vi "End Print.vi"(8 "error in (no error)":errorcluster, 11 "Stage Actor.lvlib:Stage.lvclass":refnum<class "Stage.lvclass">) -> (0 "error out":errorcluster, 3 "Actor out":refnum<class "Actor.lvclass">)   [LabVIEW 2018, in "Stage Actor.lvlib" / "Stage.lvclass"]
uses:
  Stage.lvclass
  <vilib>/ActorFramework/Actor/Actor.lvclass
  C:/Program Files/National Instruments/LabVIEW 2018/vi.lib/ActorFramework/Actor/Actor.lvclass
  Stage.lvclass/Stage.ctl
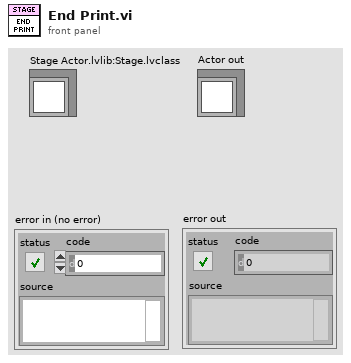
[diagram p1: front panel]
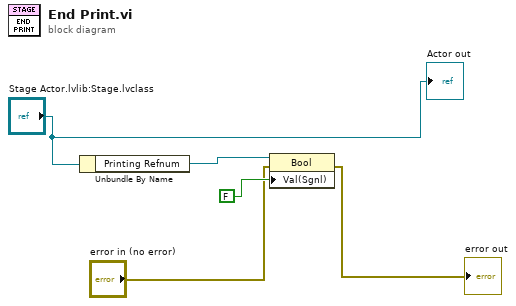
[diagram p0: block diagram]
diagram:
  n1 = Unbundle By Name("Stage Actor.lvlib:Stage.lvclass") -> ("Printing Refnum"=w5:refnum<vi>)
  n2 = property class="Bool"(reference=w5, error in="error in (no error)", "Val(Sgnl)"=FALSE) -> (error out=→"error out":errorcluster)  [unwired: 1 out]
  "Actor out" <- "Stage Actor.lvlib:Stage.lvclass"
